vi "Pockels Cal-Emergency cal source.vi"() -> (2 "SINGLE CAL SET (inc. headers & info)":string[][](array[string]))   [LabVIEW 2013]
panel:
  out "Current wavelength":dbl
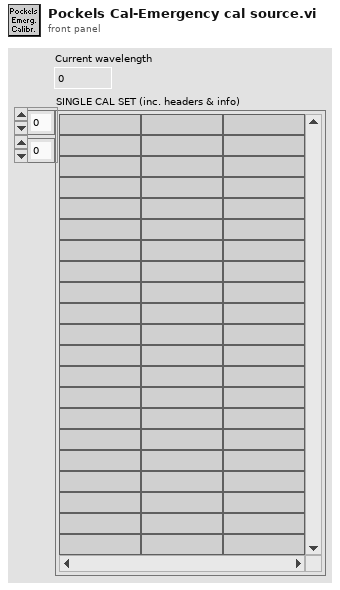
[diagram p1: front panel]
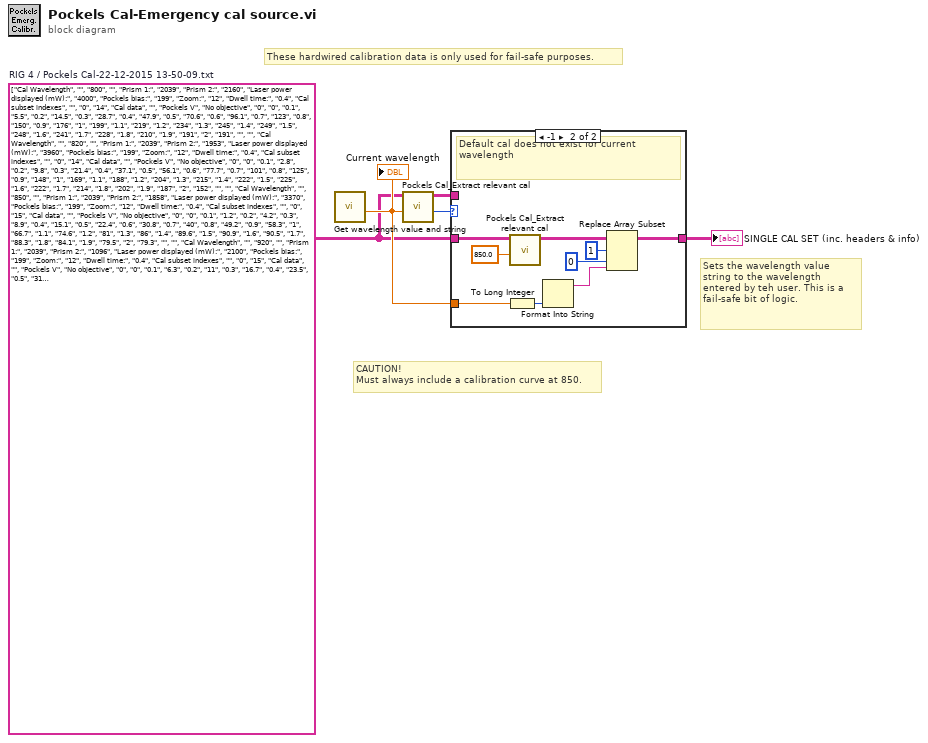
[diagram p0: block diagram]
diagram:
  w1 = string[][] [["Cal Wavelength", ""], ["800", ""], ["Prism 1:", "2039"], ["Prism 2:", "2160"], ["Laser power displayed (mW):", "4000"], ["Pockels bias:", "199"], ["Zoom:", "12"], ["Dwell time:", "0.4"], ["Cal subset indexes", ""], ["0", "14"], ["Cal data", ""], ["Pockels V", "No objective"], ["0", "0"], ["0.1", "5.5"], ["0.2", "14.5"], ["0.3", "28.7"], ["0.4", "47.9"], ["0.5", "70.6"], ["0.6", "96.1"], ["0.7", "123"], ["0.8", "150"], ["0.9", "176"], ["1", "199"], ["1.1", "219"], ["1.2", "234"], ["1.3", "245"], ["1.4", "249"], ["1.5", "248"], ["1.6", "241"], ["1.7", "228"], ["1.8", "210"], ["1.9", "191"], ["2", "191"], ["", ""], ["Cal Wavelength", ""], ["820", ""], ["Prism 1:", "2039"], ["Prism 2:", "1953"], ["Laser power displayed (mW):", "3960"], ["Pockels bias:", "199"], ["Zoom:", "12"], ["Dwell time:", "0.4"], ["Cal subset indexes", ""], ["0", "14"], ["Cal data", ""], ["Pockels V", "No objective"], ["0", "0"], ["0.1", "2.8"], ["0.2", "9.8"], ["0.3", "21.4"], ["0.4", "37.1"], ["0.5", "56.1"], ["0.6", "77.7"], ["0.7", "101"], ["0.8", "125"], ["0.9", "148"], ["1", "169"], ["1.1", "188"], ["1.2", "204"], ["1.3", "215"], ["1.4", "222"], ["1.5", "225"], ["1.6", "222"], ["1.7", "214"], ["1.8", "202"], ["1.9", "187"], ["2", "152"], ["", ""], ["Cal Wavelength", ""], ["850", ""], ["Prism 1:", "2039"], ["Prism 2:", "1858"], ["Laser power displayed (mW):", "3370"], ["Pockels bias:", "199"], ["Zoom:", "12"], ["Dwell time:", "0.4"], ["Cal subset indexes", ""], ["0", "15"], ["Cal data", ""], ["Pockels V", "No objective"], ["0", "0"], ["0.1", "1.2"], ["0.2", "4.2"], ["0.3", "8.9"], ["0.4", "15.1"], ["0.5", "22.4"], ["0.6", "30.8"], ["0.7", "40"], ["0.8", "49.2"], ["0.9", "58.3"], ["1", "66.7"], ["1.1", "74.6"], ["1.2", "81"], ["1.3", "86"], ["1.4", "89.6"], ["1.5", "90.9"], ["1.6", "90.5"], ["1.7", "88.3"], ["1.8", "84.1"], ["1.9", "79.5"], ["2", "79.3"], ["", ""], ["Cal Wavelength", ""], ["920", ""], ["Prism 1:", "2039"], ["Prism 2:", "1096"], ["Laser power displayed (mW):", "2100"], ["Pockels bias:", "199"], ["Zoom:", "12"], ["Dwell time:", "0.4"], ["Cal subset indexes", ""], ["0", "15"], ["Cal data", ""], ["Pockels V", "No objective"], ["0", "0"], ["0.1", "6.3"], ["0.2", "11"], ["0.3", "16.7"], ["0.4", "23.5"], ["0.5", "31"], ["0.6", "38.8"], ["0.7", "47"], ["0.8", "54.9"], ["0.9", "62.5"], ["1", "69.3"], ["1.1", "75.3"], ["1.2", "80"], ["1.3", "83.5"], ["1.4", "85.2"], ["1.5", "85.6"], ["1.6", "84.6"], ["1.7", "82.2"], ["1.8", "78.5"], ["1.9", "73.7"], ["2", "73.7"]]  # RIG 4 / Pockels Cal-22-12-2015 13-50-09.txt
  # "CAUTION!\nMust always include a calibration curve at 850."
  # "Sets the wavelength value string to the wavelength entered by teh user. This is a fail-safe bit of logic."
  # "These hardwired calibration data is only used for fail-safe purposes."
  n1 = call "Get wavelength value and string.vi"() -> ("Wavelength value"=w2:dbl)  [unwired: 9 in, 2 out]
  "Current wavelength" <- w2
  n2 = call "Pockels Cal_Extract relevant cal.vi"("Wavelength value"=w2, "Loaded table"=w1) -> ("Index of replacement"=w5:i32, "Relevant cal only"=w4:string[][])  [unwired: 6 in, 2 out]
  n3 = case shown="-1" w5 {
    tunnel: [w6 w8] -> w3
    tunnel: w4 -> [w6 _]
    tunnel: w1 -> [_ w11]
    tunnel: w2 -> [_ w7]
    frame Default {
      # "Defauls cal exists for the current wavelength."
    }
    frame -1 {
      # "Default cal does not exist for current wavelength"
      n4 = To Long Integer(number=w7) -> (32bit integer=w15:i32)
      n5 = call "Pockels Cal_Extract relevant cal.vi"("Wavelength value"=850.0, "Loaded table"=w11) -> ("Relevant cal only"=w10:string[][])  [unwired: 6 in, 3 out]
      n6 = Format Into String(w15) -> (resulting string=w12:string)  [unwired: 3 in, 1 out]
      n7 = Replace Array Subset(array=w10, new element=w12, index (row)=1, index (col)=0 ("disabled index (col)")) -> (w8:string[][])
    }
  }
  "SINGLE CAL SET (inc. headers & info)" <- w3
